vi "onStatusUpdated.vi"(8 "error in (no error)":errorcluster, 10 "StatusRecord":T1, 11 "CameraTestingUI in":refnum<class "CameraTestingUI.lvclass">) -> (0 "error out":errorcluster, 3 "CameraTestingUI out":refnum<class "CameraTestingUI.lvclass">)   [LabVIEW 2020, in "CameraTestingUI.lvlib" / "CameraTestingUI.lvclass"]
uses:
  CameraTestingUI.lvclass
  ICameraTesting/ICameraTesting/TypeDef/StatusRecord.ctl
  CameraTestingUI.lvclass/CameraTestingUI.ctl
  <vilib>/Utility/error.llb/DialogType.ctl
  ICameraTesting/ICameraTesting/ICameraTesting.lvclass
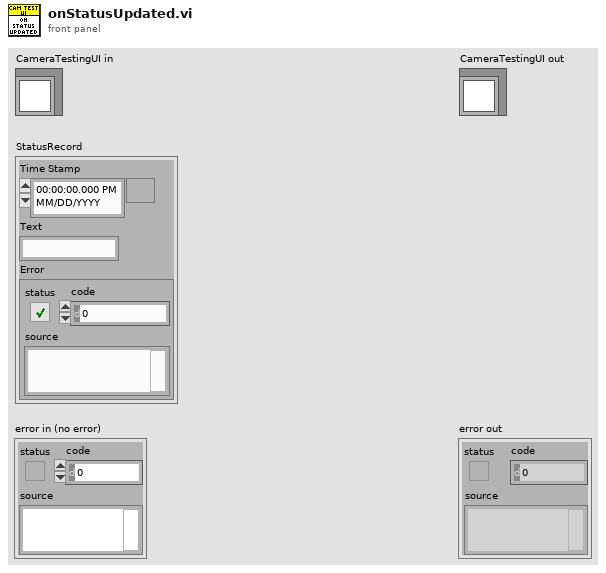
[diagram p1: front panel]
types:
  T1 = typedef "ICameraTesting.lvlib/ICameraTesting.lvclass/StatusRecord.ctl" = cluster{"Time Stamp":timestamp, "Text":string, "Error":errorcluster}
  T2 = typedef "DialogType.ctl" = u16
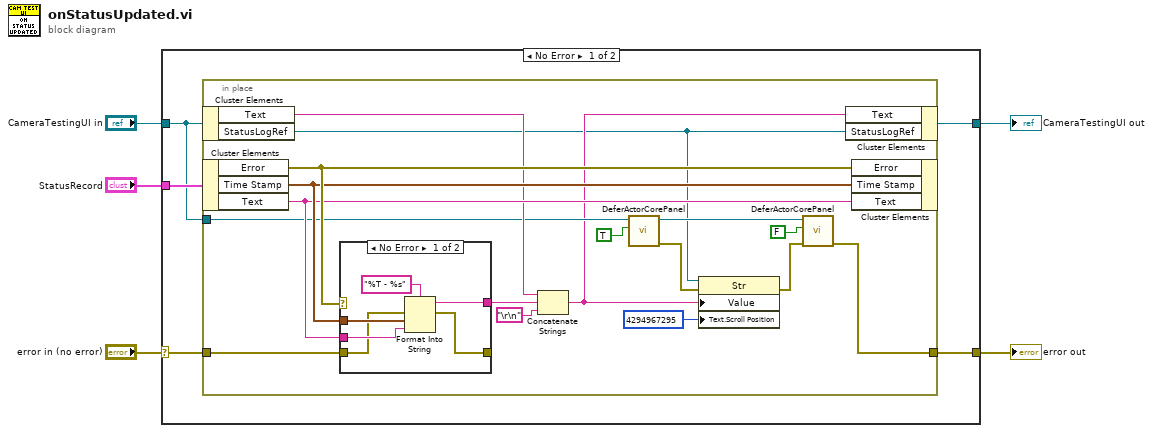
[diagram p0: block diagram]
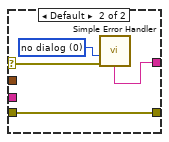
[diagram p2: hidden frame]
diagram:
  n1 = case shown="No Error" "error in (no error)" {
    selector: "error in (no error)" -> [w9 w39]
    tunnel: [w7 w39] -> w4
    tunnel: [w6 w38] -> w2
    tunnel: "CameraTestingUI in" -> [w8 w38]
    tunnel: "StatusRecord" -> [w10 _]
    frame No Error {
      n2 = in-place {
        in-place-border: w9 -> [w27]
        in-place-border: w8 -> [w14]
        in-place-border: [w11] -> w7
        n3 = in-place-cluster #1(w8) -> ("Text"=w23:string, "StatusLogRef"=w12:refnum<vi>)
        n4 = in-place-cluster #2(w10) -> ("Error"=w26:errorcluster, "Time Stamp"=w25:timestamp, "Text"=w24:string)
        n5 = case shown="No Error" w26 {
          selector: w26 -> [_ w36]
          tunnel: [w30 w34] -> w22
          tunnel: w25 -> [w32 _]
          tunnel: w24 -> [w31 _]
          tunnel: w27 -> [w29 w35]
          tunnel: [w28 w35] -> _
          frame No Error {
            n6 = Format Into String(format string="%T - %s", error in=w29, w32, w31) -> (resulting string=w30:string, error out=w28:errorcluster)  [unwired: 1 in]
          }
          frame Default {
            w37 = T2 0 items=["no dialog", "OK message", "continue or stop message", "OK message + warnings", "continue/stop + warnings"] ("type of dialog (OK msg:1)")
            n7 = call <vilib>:"Simple Error Handler.vi"("type of dialog (OK msg:1)"=w37, "error in (no error)"=w36) -> ("message"=w34:string)  [unwired: 3 in, 4 out]
          }
        }
        n8 = Concatenate Strings(w23, w22, "\r\n") -> (w13:string)
        n9 = call "DeferActorCorePanel.vi"("On/Off"=TRUE, "CameraTestingUI in"=w14) -> ("error out"=w20:errorcluster, "CameraTestingUI out"=w18:refnum<class "CameraTestingUI.lvclass">)  [unwired: 8 in]
        n10 = property class="Str"(reference=w12, error in=w20, "Value"=w13, "Text.Scroll Position"=u32 4294967295) -> (error out=w19:errorcluster)  [unwired: 1 out]
        n11 = call "DeferActorCorePanel.vi"("error in (no error)"=w19, "On/Off"=FALSE, "CameraTestingUI in"=w18) -> ("error out"=w11:errorcluster)  [unwired: 7 in, 1 out]
        n12 = in-place-cluster #1("Text"=w13, "StatusLogRef"=w12) -> (w6:refnum<class "CameraTestingUI.lvclass">)
        n13 = in-place-cluster #2("Error"=w26, "Time Stamp"=w25, "Text"=w24) -> ()  [unwired: 1 out]
      }
    }
    frame Error {
    }
  }
  "error out" <- w4
  "CameraTestingUI out" <- w2
